vi "Lab Panel V5.27.vi"() -> ()   [LabVIEW 2013] (continued)
                          frame #1 {
                            n1470 = Bundle(cluster=w2757, "STATUS"="T-RISE PASS") -> (w2759:T4)  [unwired: 2 in]
                            n1471 = local write "RESULT LAB04-1"(TRUE) -> ()
                            n1472 = local write "DISP LAB04-1"(w2759) -> ()
                          }
                        }
                      }
                      frame False {
                      }
                    }
                  }
                }
              }
              frame #7 {
                # "LAB04-2"
                n1473 = Equal?(x=w2762, y=2) -> (x = y?=w2765:bool)
                n1474 = local read "DISP LAB04-2"() -> (w2767:T4)
                n1475 = Unbundle(w2767) -> ("STATUS"=w2768:string)  [unwired: 2 out]
                n1476 = Equal?(x=w2768, y="RUN") -> (x = y?=w2764:bool)
                n1477 = And(x=w2764, y=w2765) -> (x .and. y?=w2763:bool)
                n1478 = case shown="True" w2763 {
                  tunnel: w2767 -> [_ w2771]
                  tunnel: w2761 -> [_ w2774]
                  frame False {
                  }
                  frame True {
                    n1479 = local read "SET LAB04-2"() -> (w2773:T5)
                    n1480 = local read "TDMS LAB04-2"() -> (w2770:refnum<k34>)
                    n1481 = Unbundle(w2771) -> ("CYCLE"=w2775:dbl)  [unwired: 2 out]
                    n1482 = Unbundle(w2773) -> ("T-RISE mins"=w2772:dbl)  [unwired: 4 out]
                    n1483 = Greater Or Equal?(x=w2775, y=w2774) -> (x >= y?=w2776:bool)
                    n1484 = case shown="True" w2776 {
                      tunnel: w2772 -> [w2779 _]
                      tunnel: w2771 -> [w2778 _]
                      tunnel: w2770 -> [w2777 _]
                      frame True {
                        n1485 = stacked-sequence {
                          tunnel: w2779 -> [w2782 _]
                          tunnel: w2778 -> [_ w2787]
                          tunnel: w2777 -> [w2780 _]
                          frame #0 {
                            n1486 = Build Array("T-RISE") -> (w2784:string[])
                            n1487 = Build Array(w2782) -> (w2783:dbl[])
                            n1488 = TDMS Write(0:w2780, 5:"TEST PASS", 7:w2784, 9:w2783) -> (15:w2786:errorcluster)  [unwired: 2 in, 3 out]
                            n1489 = local write "data file error"(w2786) -> ()
                          }
                          frame #1 {
                            n1490 = Bundle(cluster=w2787, "STATUS"="T-RISE PASS") -> (w2789:T4)  [unwired: 2 in]
                            n1491 = local write "RESULT LAB04-2"(TRUE) -> ()
                            n1492 = local write "DISP LAB04-2"(w2789) -> ()
                          }
                        }
                      }
                      frame False {
                      }
                    }
                  }
                }
              }
              frame #8 {
                # "LAB05-1"
                n1493 = Equal?(x=w2792, y=2) -> (x = y?=w2795:bool)
                n1494 = local read "DISP LAB05-1"() -> (w2797:T4)
                n1495 = Unbundle(w2797) -> ("STATUS"=w2798:string)  [unwired: 2 out]
                n1496 = Equal?(x=w2798, y="RUN") -> (x = y?=w2794:bool)
                n1497 = And(x=w2794, y=w2795) -> (x .and. y?=w2793:bool)
                n1498 = case shown="True" w2793 {
                  tunnel: w2797 -> [_ w2801]
                  tunnel: w2791 -> [_ w2804]
                  frame False {
                  }
                  frame True {
                    n1499 = local read "SET LAB05-1"() -> (w2803:T5)
                    n1500 = local read "TDMS LAB05-1"() -> (w2800:refnum<k34>)
                    n1501 = Unbundle(w2801) -> ("CYCLE"=w2805:dbl)  [unwired: 2 out]
                    n1502 = Unbundle(w2803) -> ("T-RISE mins"=w2802:dbl)  [unwired: 4 out]
                    n1503 = Greater Or Equal?(x=w2805, y=w2804) -> (x >= y?=w2806:bool)
                    n1504 = case shown="True" w2806 {
                      tunnel: w2802 -> [w2809 _]
                      tunnel: w2801 -> [w2808 _]
                      tunnel: w2800 -> [w2807 _]
                      frame True {
                        n1505 = stacked-sequence {
                          tunnel: w2809 -> [w2812 _]
                          tunnel: w2808 -> [_ w2817]
                          tunnel: w2807 -> [w2810 _]
                          frame #0 {
                            n1506 = Build Array("T-RISE") -> (w2814:string[])
                            n1507 = Build Array(w2812) -> (w2813:dbl[])
                            n1508 = TDMS Write(0:w2810, 5:"TEST PASS", 7:w2814, 9:w2813) -> (15:w2816:errorcluster)  [unwired: 2 in, 3 out]
                            n1509 = local write "data file error"(w2816) -> ()
                          }
                          frame #1 {
                            n1510 = Bundle(cluster=w2817, "STATUS"="T-RISE PASS") -> (w2819:T4)  [unwired: 2 in]
                            n1511 = local write "RESULT LAB05-1"(TRUE) -> ()
                            n1512 = local write "DISP LAB05-1"(w2819) -> ()
                          }
                        }
                      }
                      frame False {
                      }
                    }
                  }
                }
              }
              frame #9 {
                # "LAB05-2"
                n1513 = Equal?(x=w2822, y=2) -> (x = y?=w2825:bool)
                n1514 = local read "DISP LAB05-2"() -> (w2827:T4)
                n1515 = Unbundle(w2827) -> ("STATUS"=w2828:string)  [unwired: 2 out]
                n1516 = Equal?(x=w2828, y="RUN") -> (x = y?=w2824:bool)
                n1517 = And(x=w2824, y=w2825) -> (x .and. y?=w2823:bool)
                n1518 = case shown="True" w2823 {
                  tunnel: w2827 -> [_ w2831]
                  tunnel: w2821 -> [_ w2834]
                  frame False {
                  }
                  frame True {
                    n1519 = local read "SET LAB05-2"() -> (w2833:T5)
                    n1520 = local read "TDMS LAB05-2"() -> (w2830:refnum<k34>)
                    n1521 = Unbundle(w2831) -> ("CYCLE"=w2835:dbl)  [unwired: 2 out]
                    n1522 = Unbundle(w2833) -> ("T-RISE mins"=w2832:dbl)  [unwired: 4 out]
                    n1523 = Greater Or Equal?(x=w2835, y=w2834) -> (x >= y?=w2836:bool)
                    n1524 = case shown="True" w2836 {
                      tunnel: w2832 -> [w2839 _]
                      tunnel: w2831 -> [w2838 _]
                      tunnel: w2830 -> [w2837 _]
                      frame True {
                        n1525 = stacked-sequence {
                          tunnel: w2839 -> [w2842 _]
                          tunnel: w2838 -> [_ w2847]
                          tunnel: w2837 -> [w2840 _]
                          frame #0 {
                            n1526 = Build Array("T-RISE") -> (w2844:string[])
                            n1527 = Build Array(w2842) -> (w2843:dbl[])
                            n1528 = TDMS Write(0:w2840, 5:"TEST PASS", 7:w2844, 9:w2843) -> (15:w2846:errorcluster)  [unwired: 2 in, 3 out]
                            n1529 = local write "data file error"(w2846) -> ()
                          }
                          frame #1 {
                            n1530 = Bundle(cluster=w2847, "STATUS"="T-RISE PASS") -> (w2849:T4)  [unwired: 2 in]
                            n1531 = local write "RESULT LAB05-2"(TRUE) -> ()
                            n1532 = local write "DISP LAB05-2"(w2849) -> ()
                          }
                        }
                      }
                      frame False {
                      }
                    }
                  }
                }
              }
            }
          }
          frame #7 {
            # "end test & close test files"
            n1533 = local read "MAIL SETTINGS"() -> (w2856:T7)
            n1534 = local read "TO (string):"() -> (w2851:string)
            n1535 = Unbundle(w2856) -> ("OUT SERVER ADDRESS"=w2855:string, "FROM ACCOUNT"=w2854:string)  [unwired: 5 out]
            n1536 = stacked-sequence {
              tunnel: w2866 -> [_ _ _ _ _ _ _ _ _ _]
              tunnel: w2867 -> [_ _ _ _ _ _ _ _ _ _]
              tunnel: w2865 -> [_ _ _ _ _ _ _ _ _ _]
              tunnel: w2864 -> [_ _ _ _ _ _ _ _ _ _]
              tunnel: w2863 -> [_ _ _ _ _ _ _ _ _ _]
              tunnel: w2862 -> [_ _ _ _ _ _ _ _ _ _]
              tunnel: w2861 -> [_ _ _ _ _ _ _ _ _ _]
              tunnel: w2860 -> [_ _ _ _ _ _ _ _ _ _]
              tunnel: w2859 -> [_ _ _ _ _ _ _ _ _ _]
              tunnel: w2858 -> [_ _ _ _ _ _ _ _ _ _]
              tunnel: w2855 -> [w2872 w2923 w2971 w3018 w3065 w3112 w3159 w3206 w3253 w3300]
              tunnel: w2854 -> [w2871 w2922 w2970 w3017 w3064 w3111 w3158 w3205 w3252 w3299]
              tunnel: "Mail Test File To:" -> [w2870 w2921 w2969 w3016 w3063 w3110 w3157 w3204 w3251 w3298]
              tunnel: "Mail Test Fail" -> [w2869 w2920 w2968 w3015 w3062 w3109 w3156 w3203 w3250 w3297]
              frame #0 {
                # "LAB01-1"
                n1537 = local read "DISP LAB01-1"() -> (w2868:T4)
                n1538 = global write "Global display 2.vi" "DISP LAB01-1"(w2868) -> ()
                n1539 = local read "run lab01-1"() -> (w2873:bool)
                n1540 = local read "TDMS LAB01-1"() -> (w2874:refnum<k34>)
                n1541 = Unbundle(w2868) -> ("CYCLE"=w2876:dbl, "STATUS"=w2875:string)  [unwired: 1 out]
                n1542 = case shown="True" w2873 {
                  tunnel: w2876 -> [_ w2882]
                  tunnel: w2868 -> [_ w2884]
                  tunnel: w2875 -> [_ w2881]
                  tunnel: w2874 -> [_ w2883]
                  tunnel: w2872 -> [_ w2880]
                  tunnel: w2871 -> [_ w2879]
                  tunnel: w2870 -> [_ w2878]
                  tunnel: w2869 -> [_ w2877]
                  frame False {
                  }
                  frame True {
                    n1543 = Not Equal?(x=w2881, y="RUN") -> (x != y?=w2885:bool)
                    n1544 = Greater?(x=w2882, y=2.0) -> (0:w2887:bool)
                    n1545 = And(x=w2887, y=w2885) -> (x .and. y?=w2886:bool)
                    n1546 = case shown="True" w2886 {
                      tunnel: w2884 -> [_ w2897]
                      tunnel: w2883 -> [_ w2896]
                      tunnel: w2882 -> [_ w2895]
                      tunnel: w2881 -> [_ w2894]
                      tunnel: w2880 -> [_ w2893]
                      tunnel: w2879 -> [_ w2892]
                      tunnel: w2878 -> [_ w2891]
                      tunnel: w2877 -> [_ w2890]
                      frame False {
                      }
                      frame True {
                        n1547 = stacked-sequence {
                          tunnel: w2897 -> [w2901 _ _]
                          tunnel: w2896 -> [_ w2903 _]
                          tunnel: w2895 -> [_ _ _]
                          tunnel: w2894 -> [_ _ w2909]
                          tunnel: w2893 -> [_ _ w2908]
                          tunnel: w2892 -> [_ _ w2907]
                          tunnel: w2891 -> [_ _ w2906]
                          tunnel: w2890 -> [_ _ w2905]
                          frame #0 {
                            w2898 = FALSE
                            n1548 = local write "mail control"("END") -> ()
                            n1549 = Bundle(cluster=w2901) -> (w2900:T4)  [unwired: 3 in]
                            n1550 = local write "DISP LAB01-1"(w2900) -> ()
                            n1551 = local write "O/I  LAB01-1"(w2898) -> ()
                            n1552 = local write "run lab01-1"(w2898) -> ()
                            n1553 = local write "RUN LAB01-1"(w2898) -> ()
                          }
                          frame #1 {
                            n1554 = TDMS Close(11:w2903) -> (0:w2902:errorcluster)  [unwired: 1 in, 1 out]
                            n1555 = local write "data file error"(w2902) -> ()
                          }
                          frame #2 {
                            n1556 = stacked-sequence {
                              tunnel: "LAB01-1" -> [w2911 w2913 _]
                              tunnel: w2909 -> [_ w2919 _]
                              tunnel: w2908 -> [_ w2918 _]
                              tunnel: w2907 -> [_ w2917 _]
                              tunnel: w2906 -> [_ w2916 _]
                              tunnel: w2905 -> [_ w2915 _]
                              frame #0 {
                                n1557 = call "sub vi - defrag tdms v1.vi"("panel id"=w2911) -> ("error out"=w2910:errorcluster)  [unwired: 10 in]
                                n1558 = local write "data file error"(w2910) -> ()
                              }
                              frame #1 {
                                n1559 = Bundle("STATUS"=w2919, "OUT SERVER ADDRESS"=w2918, "FROM ACCOUNT"=w2917, "Mail Test File To:"=w2916, "Mail Test Fail"=w2915) -> (w2912:T26)  [unwired: 1 in]
                                n1560 = call "Save data file (pass-fail) v5.vi"("Input Cluster"=w2912, "panel id"=w2913) -> ("network file save error"=w2914:errorcluster)  [unwired: 8 in, 1 out]
                                n1561 = local write "data file error"(w2914) -> ()
                              }
                              frame #2 {
                              }
                            }
                          }
                        }
                      }
                    }
                  }
                }
              }
              frame #1 {
                # "LAB01-2"
                n1562 = local read "run lab01-2"() -> (w2924:bool)
                n1563 = case shown="True" w2924 {
                  tunnel: w2923 -> [_ w2929]
                  tunnel: w2922 -> [_ w2928]
                  tunnel: w2921 -> [_ w2927]
                  tunnel: w2920 -> [_ w2926]
                  frame False {
                  }
                  frame True {
                    n1564 = local read "DISP LAB01-2"() -> (w2925:T4)
                    n1565 = global write "Global display 2.vi" "DISP LAB01-2"(w2925) -> ()
                    n1566 = local read "TDMS LAB01-2"() -> (w2936:refnum<k34>)
                    n1567 = Unbundle(w2925) -> ("CYCLE"=w2931:dbl, "STATUS"=w2930:string)  [unwired: 1 out]
                    n1568 = Not Equal?(x=w2930, y="RUN") -> (x != y?=w2933:bool)
                    n1569 = Greater?(x=w2931, y=2.0) -> (0:w2934:bool)
                    n1570 = And(x=w2934, y=w2933) -> (x .and. y?=w2932:bool)
                    n1571 = case shown="True" w2932 {
                      tunnel: w2925 -> [_ w2945]
                      tunnel: w2936 -> [_ w2944]
                      tunnel: w2931 -> [_ w2943]
                      tunnel: w2930 -> [_ w2942]
                      tunnel: w2929 -> [_ w2941]
                      tunnel: w2928 -> [_ w2940]
                      tunnel: w2927 -> [_ w2939]
                      tunnel: w2926 -> [_ w2938]
                      frame False {
                      }
                      frame True {
                        n1572 = stacked-sequence {
                          tunnel: w2945 -> [w2948 _ _]
                          tunnel: w2944 -> [_ w2950 _]
                          tunnel: w2943 -> [_ _ _]
                          tunnel: w2942 -> [_ _ w2956]
                          tunnel: w2941 -> [_ _ w2955]
                          tunnel: w2940 -> [_ _ w2954]
                          tunnel: w2939 -> [_ _ w2953]
                          tunnel: w2938 -> [_ _ w2952]
                          frame #0 {
                            w2946 = FALSE
                            n1573 = local write "mail control"("END") -> ()
                            n1574 = Bundle(cluster=w2948) -> (w2949:T4)  [unwired: 3 in]
                            n1575 = local write "RUN LAB01-2"(w2946) -> ()
                            n1576 = local write "run lab01-2"(w2946) -> ()
                            n1577 = local write "O/I  LAB01-2"(w2946) -> ()
                            n1578 = local write "DISP LAB01-2"(w2949) -> ()
                          }
                          frame #1 {
                            n1579 = TDMS Close(11:w2950) -> (0:w2951:errorcluster)  [unwired: 1 in, 1 out]
                            n1580 = local write "data file error"(w2951) -> ()
                          }
                          frame #2 {
                            n1581 = stacked-sequence {
                              tunnel: "LAB01-2" -> [w2959 w2960]
                              tunnel: w2956 -> [_ w2965]
                              tunnel: w2955 -> [_ w2964]
                              tunnel: w2954 -> [_ w2963]
                              tunnel: w2953 -> [_ w2962]
                              tunnel: w2952 -> [_ w2961]
                              frame #0 {
                                n1582 = call "sub vi - defrag tdms v1.vi"("panel id"=w2959) -> ("error out"=w2958:errorcluster)  [unwired: 10 in]
                                n1583 = local write "data file error"(w2958) -> ()
                              }
                              frame #1 {
                                n1584 = Bundle("STATUS"=w2965, "OUT SERVER ADDRESS"=w2964, "FROM ACCOUNT"=w2963, "Mail Test File To:"=w2962, "Mail Test Fail"=w2961) -> (w2967:T26)  [unwired: 1 in]
                                n1585 = call "Save data file (pass-fail) v5.vi"("Input Cluster"=w2967, "panel id"=w2960) -> ("network file save error"=w2966:errorcluster)  [unwired: 8 in, 1 out]
                                n1586 = local write "data file error"(w2966) -> ()
                              }
                            }
                          }
                        }
                      }
                    }
                  }
                }
              }
              frame #2 {
                # "LAB02-1"
                n1587 = local read "run lab02-1"() -> (w2972:bool)
                n1588 = case shown="True" w2972 {
                  tunnel: w2971 -> [_ w2977]
                  tunnel: w2970 -> [_ w2976]
                  tunnel: w2969 -> [_ w2975]
                  tunnel: w2968 -> [_ w2974]
                  frame False {
                  }
                  frame True {
                    n1589 = local read "DISP LAB02-1"() -> (w2973:T4)
                    n1590 = global write "Global display 2.vi" "DISP LAB02-1"(w2973) -> ()
                    n1591 = Unbundle(w2973) -> ("CYCLE"=w2981:dbl, "STATUS"=w2978:string)  [unwired: 1 out]
                    n1592 = local read "TDMS LAB02-1"() -> (w2984:refnum<k34>)
                    n1593 = Not Equal?(x=w2978, y="RUN") -> (x != y?=w2980:bool)
                    n1594 = Greater?(x=w2981, y=2.0) -> (0:w2982:bool)
                    n1595 = And(x=w2982, y=w2980) -> (x .and. y?=w2979:bool)
                    n1596 = case shown="True" w2979 {
                      tunnel: w2973 -> [_ w2992]
                      tunnel: w2984 -> [_ w2991]
                      tunnel: w2978 -> [_ w2990]
                      tunnel: w2977 -> [_ w2989]
                      tunnel: w2976 -> [_ w2988]
                      tunnel: w2975 -> [_ w2987]
                      tunnel: w2974 -> [_ w2986]
                      frame False {
                      }
                      frame True {
                        n1597 = stacked-sequence {
                          tunnel: w2992 -> [w2995 _ _]
                          tunnel: w2991 -> [_ w2997 _]
                          tunnel: w2990 -> [_ _ w3003]
                          tunnel: w2989 -> [_ _ w3002]
                          tunnel: w2988 -> [_ _ w3001]
                          tunnel: w2987 -> [_ _ w3000]
                          tunnel: w2986 -> [_ _ w2999]
                          frame #0 {
                            w2993 = FALSE
                            n1598 = local write "mail control"("END") -> ()
                            n1599 = Bundle(cluster=w2995) -> (w2996:T4)  [unwired: 3 in]
                            n1600 = local write "O/I  LAB02-1"(w2993) -> ()
                            n1601 = local write "RUN LAB02-1"(w2993) -> ()
                            n1602 = local write "run lab02-1"(w2993) -> ()
                            n1603 = local write "DISP LAB02-1"(w2996) -> ()
                          }
                          frame #1 {
                            n1604 = TDMS Close(11:w2997) -> (0:w2998:errorcluster)  [unwired: 1 in, 1 out]
                            n1605 = local write "data file error"(w2998) -> ()
                          }
                          frame #2 {
                            n1606 = stacked-sequence {
                              tunnel: "LAB02-1" -> [w3006 w3013]
                              tunnel: w3003 -> [_ w3011]
                              tunnel: w3002 -> [_ w3010]
                              tunnel: w3001 -> [_ w3009]
                              tunnel: w3000 -> [_ w3008]
                              tunnel: w2999 -> [_ w3007]
                              frame #0 {
                                n1607 = call "sub vi - defrag tdms v1.vi"("panel id"=w3006) -> ("error out"=w3005:errorcluster)  [unwired: 10 in]
                                n1608 = local write "data file error"(w3005) -> ()
                              }
                              frame #1 {
                                n1609 = Bundle("STATUS"=w3011, "OUT SERVER ADDRESS"=w3010, "FROM ACCOUNT"=w3009, "Mail Test File To:"=w3008, "Mail Test Fail"=w3007) -> (w3012:T26)  [unwired: 1 in]
                                n1610 = call "Save data file (pass-fail) v5.vi"("Input Cluster"=w3012, "panel id"=w3013) -> ("network file save error"=w3014:errorcluster)  [unwired: 8 in, 1 out]
                                n1611 = local write "data file error"(w3014) -> ()
                              }
                            }
                          }
                        }
                      }
                    }
                  }
                }
              }
              frame #3 {
                # "LAB02-2"
                n1612 = local read "run lab02-2"() -> (w3019:bool)
                n1613 = case shown="True" w3019 {
                  tunnel: w3018 -> [_ w3025]
                  tunnel: w3017 -> [_ w3024]
                  tunnel: w3016 -> [_ w3023]
                  tunnel: w3015 -> [_ w3022]
                  frame False {
                  }
                  frame True {
                    n1614 = local read "DISP LAB02-2"() -> (w3021:T4)
                    n1615 = global write "Global display 2.vi" "DISP LAB02-2"(w3021) -> ()
                    n1616 = local read "TDMS LAB02-2"() -> (w3031:refnum<k34>)
                    n1617 = Unbundle(w3021) -> ("CYCLE"=w3020:dbl, "STATUS"=w3026:string)  [unwired: 1 out]
                    n1618 = Not Equal?(x=w3026, y="RUN") -> (x != y?=w3028:bool)
                    n1619 = Greater?(x=w3020, y=2.0) -> (0:w3029:bool)
                    n1620 = And(x=w3029, y=w3028) -> (x .and. y?=w3027:bool)
                    n1621 = case shown="True" w3027 {
                      tunnel: w3021 -> [_ w3039]
                      tunnel: w3031 -> [_ w3038]
                      tunnel: w3026 -> [_ w3037]
                      tunnel: w3025 -> [_ w3036]
                      tunnel: w3024 -> [_ w3035]
                      tunnel: w3023 -> [_ w3034]
                      tunnel: w3022 -> [_ w3033]
                      frame False {
                      }
                      frame True {
                        n1622 = stacked-sequence {
                          tunnel: w3039 -> [w3042 _ _]
                          tunnel: w3038 -> [_ w3044 _]
                          tunnel: w3037 -> [_ _ w3050]
                          tunnel: w3036 -> [_ _ w3049]
                          tunnel: w3035 -> [_ _ w3048]
                          tunnel: w3034 -> [_ _ w3047]
                          tunnel: w3033 -> [_ _ w3046]
                          frame #0 {
                            w3040 = FALSE
                            n1623 = local write "mail control"("END") -> ()
                            n1624 = Bundle(cluster=w3042) -> (w3043:T4)  [unwired: 3 in]
                            n1625 = local write "O/I  LAB02-2"(w3040) -> ()
                            n1626 = local write "run lab02-2"(w3040) -> ()
                            n1627 = local write "RUN LAB02-2"(w3040) -> ()
                            n1628 = local write "DISP LAB02-2"(w3043) -> ()
                          }
                          frame #1 {
                            n1629 = TDMS Close(11:w3044) -> (0:w3045:errorcluster)  [unwired: 1 in, 1 out]
                            n1630 = local write "data file error"(w3045) -> ()
                          }
                          frame #2 {
                            n1631 = stacked-sequence {
                              tunnel: "LAB02-2" -> [w3053 w3059]
                              tunnel: w3050 -> [_ w3058]
                              tunnel: w3049 -> [_ w3057]
                              tunnel: w3048 -> [_ w3056]
                              tunnel: w3047 -> [_ w3055]
                              tunnel: w3046 -> [_ w3054]
                              frame #0 {
                                n1632 = call "sub vi - defrag tdms v1.vi"("panel id"=w3053) -> ("error out"=w3052:errorcluster)  [unwired: 10 in]
                                n1633 = local write "data file error"(w3052) -> ()
                              }
                              frame #1 {
                                n1634 = Bundle("STATUS"=w3058, "OUT SERVER ADDRESS"=w3057, "FROM ACCOUNT"=w3056, "Mail Test File To:"=w3055, "Mail Test Fail"=w3054) -> (w3061:T26)  [unwired: 1 in]
                                n1635 = call "Save data file (pass-fail) v5.vi"("Input Cluster"=w3061, "panel id"=w3059) -> ("network file save error"=w3060:errorcluster)  [unwired: 8 in, 1 out]
                                n1636 = local write "data file error"(w3060) -> ()
                              }
                            }
                          }
                        }
                      }
                    }
                  }
                }
              }
              frame #4 {
                # "LAB03-1"
                n1637 = local read "run lab03-1"() -> (w3066:bool)
                n1638 = case shown="True" w3066 {
                  tunnel: w3065 -> [_ w3071]
                  tunnel: w3064 -> [_ w3070]
                  tunnel: w3063 -> [_ w3069]
                  tunnel: w3062 -> [_ w3068]
                  frame False {
                  }
                  frame True {
                    n1639 = local read "DISP LAB03-1"() -> (w3067:T4)
                    n1640 = local read "TDMS LAB03-1"() -> (w3078:refnum<k34>)
                    n1641 = global write "Global display 2.vi" "DISP LAB03-1"(w3067) -> ()
                    n1642 = Unbundle(w3067) -> ("CYCLE"=w3075:dbl, "STATUS"=w3072:string)  [unwired: 1 out]
                    n1643 = Not Equal?(x=w3072, y="RUN") -> (x != y?=w3074:bool)
                    n1644 = Greater?(x=w3075, y=2.0) -> (0:w3076:bool)
                    n1645 = And(x=w3076, y=w3074) -> (x .and. y?=w3073:bool)
                    n1646 = case shown="True" w3073 {
                      tunnel: w3067 -> [_ w3086]
                      tunnel: w3078 -> [_ w3085]
                      tunnel: w3072 -> [_ w3084]
                      tunnel: w3071 -> [_ w3083]
                      tunnel: w3070 -> [_ w3082]
                      tunnel: w3069 -> [_ w3081]
                      tunnel: w3068 -> [_ w3080]
                      frame False {
                      }
                      frame True {
                        n1647 = stacked-sequence {
                          tunnel: w3086 -> [w3089 _ _]
                          tunnel: w3085 -> [_ w3091 _]
                          tunnel: w3084 -> [_ _ w3097]
                          tunnel: w3083 -> [_ _ w3096]
                          tunnel: w3082 -> [_ _ w3095]
                          tunnel: w3081 -> [_ _ w3094]
                          tunnel: w3080 -> [_ _ w3093]
                          frame #0 {
                            w3087 = FALSE
                            n1648 = local write "mail control"("END") -> ()
                            n1649 = Bundle(cluster=w3089) -> (w3090:T4)  [unwired: 3 in]
                            n1650 = local write "O/I  LAB03-1"(w3087) -> ()
                            n1651 = local write "run lab03-1"(w3087) -> ()
                            n1652 = local write "RUN LAB03-1"(w3087) -> ()
                            n1653 = local write "DISP LAB03-1"(w3090) -> ()
                          }
                          frame #1 {
                            n1654 = TDMS Close(11:w3091) -> (0:w3092:errorcluster)  [unwired: 1 in, 1 out]
                            n1655 = local write "data file error"(w3092) -> ()
                          }
                          frame #2 {
                            n1656 = stacked-sequence {
                              tunnel: "LAB03-1" -> [w3100 w3106]
                              tunnel: w3097 -> [_ w3105]
                              tunnel: w3096 -> [_ w3104]
                              tunnel: w3095 -> [_ w3103]
                              tunnel: w3094 -> [_ w3102]
                              tunnel: w3093 -> [_ w3101]
                              frame #0 {
                                n1657 = call "sub vi - defrag tdms v1.vi"("panel id"=w3100) -> ("error out"=w3099:errorcluster)  [unwired: 10 in]
                                n1658 = local write "data file error"(w3099) -> ()
                              }
                              frame #1 {
                                n1659 = Bundle("STATUS"=w3105, "OUT SERVER ADDRESS"=w3104, "FROM ACCOUNT"=w3103, "Mail Test File To:"=w3102, "Mail Test Fail"=w3101) -> (w3108:T26)  [unwired: 1 in]
                                n1660 = call "Save data file (pass-fail) v5.vi"("Input Cluster"=w3108, "panel id"=w3106) -> ("network file save error"=w3107:errorcluster)  [unwired: 8 in, 1 out]
                                n1661 = local write "data file error"(w3107) -> ()
                              }
                            }
                          }
                        }
                      }
                    }
                  }
                }
              }
              frame #5 {
                # "LAB03-2"
                n1662 = local read "run lab03-2"() -> (w3113:bool)
                n1663 = case shown="True" w3113 {
                  tunnel: w3112 -> [_ w3118]
                  tunnel: w3111 -> [_ w3117]
                  tunnel: w3110 -> [_ w3116]
                  tunnel: w3109 -> [_ w3115]
                  frame False {
                  }
                  frame True {
                    n1664 = local read "DISP LAB03-2"() -> (w3114:T4)
                    n1665 = global write "Global display 2.vi" "DISP LAB03-2"(w3114) -> ()
                    n1666 = Unbundle(w3114) -> ("CYCLE"=w3122:dbl, "STATUS"=w3119:string)  [unwired: 1 out]
                    n1667 = local read "TDMS LAB03-2"() -> (w3125:refnum<k34>)
                    n1668 = Not Equal?(x=w3119, y="RUN") -> (x != y?=w3121:bool)
                    n1669 = Greater?(x=w3122, y=2.0) -> (0:w3123:bool)
                    n1670 = And(x=w3123, y=w3121) -> (x .and. y?=w3120:bool)
                    n1671 = case shown="True" w3120 {
                      tunnel: w3114 -> [_ w3133]
                      tunnel: w3125 -> [_ w3132]
                      tunnel: w3119 -> [_ w3131]
                      tunnel: w3118 -> [_ w3130]
                      tunnel: w3117 -> [_ w3129]
                      tunnel: w3116 -> [_ w3128]
                      tunnel: w3115 -> [_ w3127]
                      frame False {
                      }
                      frame True {
                        n1672 = stacked-sequence {
                          tunnel: w3133 -> [w3136 _ _]
                          tunnel: w3132 -> [_ w3138 _]
                          tunnel: w3131 -> [_ _ w3144]
                          tunnel: w3130 -> [_ _ w3143]
                          tunnel: w3129 -> [_ _ w3142]
                          tunnel: w3128 -> [_ _ w3141]
                          tunnel: w3127 -> [_ _ w3140]
                          frame #0 {
                            w3134 = FALSE
                            n1673 = local write "mail control"("END") -> ()
                            n1674 = Bundle(cluster=w3136) -> (w3137:T4)  [unwired: 3 in]
                            n1675 = local write "RUN LAB03-2"(w3134) -> ()
                            n1676 = local write "O/I  LAB03-2"(w3134) -> ()
                            n1677 = local write "DISP LAB03-2"(w3137) -> ()
                            n1678 = local write "run lab03-2"(w3134) -> ()
                          }
                          frame #1 {
                            n1679 = TDMS Close(11:w3138) -> (0:w3139:errorcluster)  [unwired: 1 in, 1 out]
                            n1680 = local write "data file error"(w3139) -> ()
                          }
                          frame #2 {
                            n1681 = stacked-sequence {
                              tunnel: "LAB03-2" -> [w3147 w3148]
                              tunnel: w3144 -> [_ w3153]
                              tunnel: w3143 -> [_ w3152]
                              tunnel: w3142 -> [_ w3151]
                              tunnel: w3141 -> [_ w3150]
                              tunnel: w3140 -> [_ w3149]
                              frame #0 {
                                n1682 = call "sub vi - defrag tdms v1.vi"("panel id"=w3147) -> ("error out"=w3146:errorcluster)  [unwired: 10 in]
                                n1683 = local write "data file error"(w3146) -> ()
                              }
                              frame #1 {
                                n1684 = Bundle("STATUS"=w3153, "OUT SERVER ADDRESS"=w3152, "FROM ACCOUNT"=w3151, "Mail Test File To:"=w3150, "Mail Test Fail"=w3149) -> (w3155:T26)  [unwired: 1 in]
                                n1685 = call "Save data file (pass-fail) v5.vi"("Input Cluster"=w3155, "panel id"=w3148) -> ("network file save error"=w3154:errorcluster)  [unwired: 8 in, 1 out]
                                n1686 = local write "data file error"(w3154) -> ()
                              }
                            }
                          }
                        }
                      }
                    }
                  }
                }
              }
              frame #6 {
                # "LAB04-1"
                n1687 = local read "run lab04-1"() -> (w3160:bool)
                n1688 = case shown="True" w3160 {
                  tunnel: w3159 -> [_ w3165]
                  tunnel: w3158 -> [_ w3164]
                  tunnel: w3157 -> [_ w3163]
                  tunnel: w3156 -> [_ w3162]
                  frame False {
                  }
                  frame True {
                    n1689 = local read "DISP LAB04-1"() -> (w3161:T4)
                    n1690 = Unbundle(w3161) -> ("CYCLE"=w3169:dbl, "STATUS"=w3166:string)  [unwired: 1 out]
                    n1691 = local read "TDMS LAB04-1"() -> (w3172:refnum<k34>)
                    n1692 = global write "Global display 2.vi" "DISP LAB04-1"(w3161) -> ()
                    n1693 = Not Equal?(x=w3166, y="RUN") -> (x != y?=w3168:bool)
                    n1694 = Greater?(x=w3169, y=2.0) -> (0:w3170:bool)
                    n1695 = And(x=w3170, y=w3168) -> (x .and. y?=w3167:bool)
                    n1696 = case shown="True" w3167 {
                      tunnel: w3161 -> [_ w3180]
                      tunnel: w3172 -> [_ w3179]
                      tunnel: w3166 -> [_ w3178]
                      tunnel: w3165 -> [_ w3177]
                      tunnel: w3164 -> [_ w3176]
                      tunnel: w3163 -> [_ w3175]
                      tunnel: w3162 -> [_ w3174]
                      frame False {
                      }
                      frame True {
                        n1697 = stacked-sequence {
                          tunnel: w3180 -> [w3183 _ _]
                          tunnel: w3179 -> [_ w3185 _]
                          tunnel: w3178 -> [_ _ w3191]
                          tunnel: w3177 -> [_ _ w3190]
                          tunnel: w3176 -> [_ _ w3189]
                          tunnel: w3175 -> [_ _ w3188]
                          tunnel: w3174 -> [_ _ w3187]
                          frame #0 {
                            w3181 = FALSE
                            n1698 = local write "mail control"("END") -> ()
                            n1699 = Bundle(cluster=w3183) -> (w3184:T4)  [unwired: 3 in]
                            n1700 = local write "RUN LAB04-1"(w3181) -> ()
                            n1701 = local write "O/I  LAB04-1"(w3181) -> ()
                            n1702 = local write "run lab04-1"(w3181) -> ()
                            n1703 = local write "DISP LAB04-1"(w3184) -> ()
                          }
                          frame #1 {
                            n1704 = TDMS Close(11:w3185) -> (0:w3186:errorcluster)  [unwired: 1 in, 1 out]
                            n1705 = local write "data file error"(w3186) -> ()
                          }
                          frame #2 {
                            n1706 = stacked-sequence {
                              tunnel: "LAB04-1" -> [w3194 w3195]
                              tunnel: w3191 -> [_ w3200]
                              tunnel: w3190 -> [_ w3199]
                              tunnel: w3189 -> [_ w3198]
                              tunnel: w3188 -> [_ w3197]
                              tunnel: w3187 -> [_ w3196]
                              frame #0 {
                                n1707 = call "sub vi - defrag tdms v1.vi"("panel id"=w3194) -> ("error out"=w3193:errorcluster)  [unwired: 10 in]
                                n1708 = local write "data file error"(w3193) -> ()
                              }
                              frame #1 {
                                n1709 = Bundle("STATUS"=w3200, "OUT SERVER ADDRESS"=w3199, "FROM ACCOUNT"=w3198, "Mail Test File To:"=w3197, "Mail Test Fail"=w3196) -> (w3202:T26)  [unwired: 1 in]
                                n1710 = call "Save data file (pass-fail) v5.vi"("Input Cluster"=w3202, "panel id"=w3195) -> ("network file save error"=w3201:errorcluster)  [unwired: 8 in, 1 out]
                                n1711 = local write "data file error"(w3201) -> ()
                              }
                            }
                          }
                        }
                      }
                    }
                  }
                }
              }
              frame #7 {
                # "LAB04-2"
                n1712 = local read "run lab04-2"() -> (w3207:bool)
                n1713 = case shown="True" w3207 {
                  tunnel: w3206 -> [_ w3212]
                  tunnel: w3205 -> [_ w3211]
                  tunnel: w3204 -> [_ w3210]
                  tunnel: w3203 -> [_ w3209]
                  frame False {
                  }
                  frame True {
                    n1714 = local read "DISP LAB04-2"() -> (w3208:T4)
                    n1715 = Unbundle(w3208) -> ("CYCLE"=w3216:dbl, "STATUS"=w3213:string)  [unwired: 1 out]
                    n1716 = global write "Global display 2.vi" "DISP LAB04-2"(w3208) -> ()
                    n1717 = Not Equal?(x=w3213, y="RUN") -> (x != y?=w3215:bool)
                    n1718 = local read "TDMS LAB04-2"() -> (w3219:refnum<k34>)
                    n1719 = Greater?(x=w3216, y=2.0) -> (0:w3217:bool)
                    n1720 = And(x=w3217, y=w3215) -> (x .and. y?=w3214:bool)
                    n1721 = case shown="True" w3214 {
                      tunnel: w3208 -> [_ w3227]
                      tunnel: w3219 -> [_ w3226]
                      tunnel: w3213 -> [_ w3225]
                      tunnel: w3212 -> [_ w3224]
                      tunnel: w3211 -> [_ w3223]
                      tunnel: w3210 -> [_ w3222]
                      tunnel: w3209 -> [_ w3221]
                      frame False {
                      }
                      frame True {
                        n1722 = stacked-sequence {
                          tunnel: w3227 -> [w3230 _ _]
                          tunnel: w3226 -> [_ w3232 _]
                          tunnel: w3225 -> [_ _ w3238]
                          tunnel: w3224 -> [_ _ w3237]
                          tunnel: w3223 -> [_ _ w3236]
                          tunnel: w3222 -> [_ _ w3235]
                          tunnel: w3221 -> [_ _ w3234]
                          frame #0 {
                            w3228 = FALSE
                            n1723 = local write "mail control"("END") -> ()
                            n1724 = Bundle(cluster=w3230) -> (w3231:T4)  [unwired: 3 in]
                            n1725 = local write "O/I  LAB04-2"(w3228) -> ()
                            n1726 = local write "RUN LAB04-2"(w3228) -> ()
                            n1727 = local write "run lab04-2"(w3228) -> ()
                            n1728 = local write "DISP LAB04-2"(w3231) -> ()
                          }
                          frame #1 {
                            n1729 = TDMS Close(11:w3232) -> (0:w3233:errorcluster)  [unwired: 1 in, 1 out]
                            n1730 = local write "data file error"(w3233) -> ()
                          }
                          frame #2 {
                            n1731 = stacked-sequence {
                              tunnel: "LAB04-2" -> [w3241 w3242]
                              tunnel: w3238 -> [_ w3247]
                              tunnel: w3237 -> [_ w3246]
                              tunnel: w3236 -> [_ w3245]
                              tunnel: w3235 -> [_ w3244]
                              tunnel: w3234 -> [_ w3243]
                              frame #0 {
                                n1732 = call "sub vi - defrag tdms v1.vi"("panel id"=w3241) -> ("error out"=w3240:errorcluster)  [unwired: 10 in]
                                n1733 = local write "data file error"(w3240) -> ()
                              }
                              frame #1 {
                                n1734 = Bundle("STATUS"=w3247, "OUT SERVER ADDRESS"=w3246, "FROM ACCOUNT"=w3245, "Mail Test File To:"=w3244, "Mail Test Fail"=w3243) -> (w3249:T26)  [unwired: 1 in]
                                n1735 = call "Save data file (pass-fail) v5.vi"("Input Cluster"=w3249, "panel id"=w3242) -> ("network file save error"=w3248:errorcluster)  [unwired: 8 in, 1 out]
                                n1736 = local write "data file error"(w3248) -> ()
                              }
                            }
                          }
                        }
                      }
                    }
                  }
                }
              }
              frame #8 {
                # "LAB05-1"
                n1737 = local read "run lab05-1"() -> (w3254:bool)
                n1738 = case shown="True" w3254 {
                  tunnel: w3253 -> [_ w3259]
                  tunnel: w3252 -> [_ w3258]
                  tunnel: w3251 -> [_ w3257]
                  tunnel: w3250 -> [_ w3256]
                  frame False {
                  }
                  frame True {
                    n1739 = local read "DISP LAB05-1"() -> (w3255:T4)
                    n1740 = Unbundle(w3255) -> ("CYCLE"=w3263:dbl, "STATUS"=w3260:string)  [unwired: 1 out]
                    n1741 = global write "Global display 2.vi" "DISP LAB05-1"(w3255) -> ()
                    n1742 = Not Equal?(x=w3260, y="RUN") -> (x != y?=w3262:bool)
                    n1743 = local read "TDMS LAB05-1"() -> (w3266:refnum<k34>)
                    n1744 = Greater?(x=w3263, y=2.0) -> (0:w3264:bool)
                    n1745 = And(x=w3264, y=w3262) -> (x .and. y?=w3261:bool)
                    n1746 = case shown="True" w3261 {
                      tunnel: w3255 -> [_ w3274]
                      tunnel: w3266 -> [_ w3273]
                      tunnel: w3260 -> [_ w3272]
                      tunnel: w3259 -> [_ w3271]
                      tunnel: w3258 -> [_ w3270]
                      tunnel: w3257 -> [_ w3269]
                      tunnel: w3256 -> [_ w3268]
                      frame False {
                      }
                      frame True {
                        n1747 = stacked-sequence {
                          tunnel: w3274 -> [w3277 _ _]
                          tunnel: w3273 -> [_ w3279 _]
                          tunnel: w3272 -> [_ _ w3285]
                          tunnel: w3271 -> [_ _ w3284]
                          tunnel: w3270 -> [_ _ w3283]
                          tunnel: w3269 -> [_ _ w3282]
                          tunnel: w3268 -> [_ _ w3281]
                          frame #0 {
                            w3275 = FALSE
                            n1748 = local write "mail control"("END") -> ()
                            n1749 = Bundle(cluster=w3277) -> (w3278:T4)  [unwired: 3 in]
                            n1750 = local write "O/I  LAB05-1"(w3275) -> ()
                            n1751 = local write "RUN LAB05-1"(w3275) -> ()
                            n1752 = local write "run lab05-1"(w3275) -> ()
                            n1753 = local write "DISP LAB05-1"(w3278) -> ()
                          }
                          frame #1 {
                            n1754 = TDMS Close(11:w3279) -> (0:w3280:errorcluster)  [unwired: 1 in, 1 out]
                            n1755 = local write "data file error"(w3280) -> ()
                          }
                          frame #2 {
                            n1756 = stacked-sequence {
                              tunnel: "LAB05-1" -> [w3288 w3294]
                              tunnel: w3285 -> [_ w3293]
                              tunnel: w3284 -> [_ w3292]
                              tunnel: w3283 -> [_ w3291]
                              tunnel: w3282 -> [_ w3290]
                              tunnel: w3281 -> [_ w3289]
                              frame #0 {
                                n1757 = call "sub vi - defrag tdms v1.vi"("panel id"=w3288) -> ("error out"=w3287:errorcluster)  [unwired: 10 in]
                                n1758 = local write "data file error"(w3287) -> ()
                              }
                              frame #1 {
                                n1759 = Bundle("STATUS"=w3293, "OUT SERVER ADDRESS"=w3292, "FROM ACCOUNT"=w3291, "Mail Test File To:"=w3290, "Mail Test Fail"=w3289) -> (w3296:T26)  [unwired: 1 in]
                                n1760 = call "Save data file (pass-fail) v5.vi"("Input Cluster"=w3296, "panel id"=w3294) -> ("network file save error"=w3295:errorcluster)  [unwired: 8 in, 1 out]
                                n1761 = local write "data file error"(w3295) -> ()
                              }
                            }
                          }
                        }
                      }
                    }
                  }
                }
              }
              frame #9 {
                # "LAB05-2"
                n1762 = local read "run lab05-2"() -> (w3301:bool)
                n1763 = case shown="True" w3301 {
                  tunnel: w3300 -> [_ w3306]
                  tunnel: w3299 -> [_ w3305]
                  tunnel: w3298 -> [_ w3304]
                  tunnel: w3297 -> [_ w3303]
                  frame False {
                  }
                  frame True {
                    n1764 = local read "DISP LAB05-2"() -> (w3302:T4)
                    n1765 = Unbundle(w3302) -> ("CYCLE"=w3310:dbl, "STATUS"=w3307:string)  [unwired: 1 out]
                    n1766 = global write "Global display 2.vi" "DISP LAB05-2"(w3302) -> ()
                    n1767 = Not Equal?(x=w3307, y="RUN") -> (x != y?=w3309:bool)
                    n1768 = local read "TDMS LAB05-2"() -> (w3313:refnum<k34>)
                    n1769 = Greater?(x=w3310, y=2.0) -> (0:w3311:bool)
                    n1770 = And(x=w3311, y=w3309) -> (x .and. y?=w3308:bool)
                    n1771 = case shown="True" w3308 {
                      tunnel: w3302 -> [_ w3321]
                      tunnel: w3313 -> [_ w3320]
                      tunnel: w3307 -> [_ w3319]
                      tunnel: w3306 -> [_ w3318]
                      tunnel: w3305 -> [_ w3317]
                      tunnel: w3304 -> [_ w3316]
                      tunnel: w3303 -> [_ w3315]
                      frame False {
                      }
                      frame True {
                        n1772 = stacked-sequence {
                          tunnel: w3321 -> [w3324 _ _]
                          tunnel: w3320 -> [_ w3326 _]
                          tunnel: w3319 -> [_ _ w3332]
                          tunnel: w3318 -> [_ _ w3331]
                          tunnel: w3317 -> [_ _ w3330]
                          tunnel: w3316 -> [_ _ w3329]
                          tunnel: w3315 -> [_ _ w3328]
                          frame #0 {
                            w3322 = FALSE
                            n1773 = local write "mail control"("END") -> ()
